vi "Remove Conditional Disable Structure.vi"(8 "error in (no error)":errorcluster, 11 "Assert VI Path":path) -> (0 "error out":errorcluster)   [LabVIEW 2018, in "Test.lvclass"]
uses:
  Test.lvclass
  <vilib>/Utility/traverseref.llb/TRef TravTarget.ctl
  Save VI Ref Source.ctl
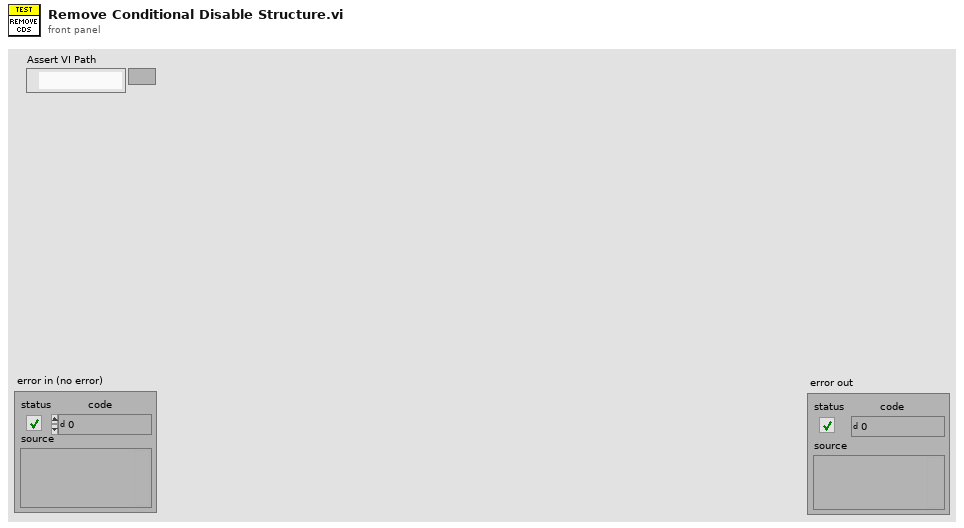
[diagram p1: front panel]
types:
  T1 = typedef "Save VI Ref Source.ctl" = enum16{"File Path", "VI Reference"}
  T2 = typedef "TRef TravTarget.ctl" = enum16{"FP", "BD", "Other"}
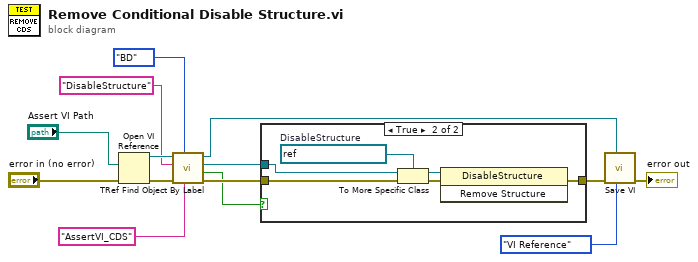
[diagram p0: block diagram]
diagram:
  n1 = Open VI Reference(vi path="Assert VI Path", error in (no error)="error in (no error)") -> (vi reference=w14:refnum<vi>, error out=w13:errorcluster)  [unwired: 4 in]
  n2 = call <vilib>:"TRef Find Object By Label.vi"("Label"="AssertVI_CDS" ("Class Name"), "Traverse Target"=TRef_TravTarget."BD", "error in (no error)"=w13, "Class Name"="DisableStructure", "VI Ref"=w14) -> ("error out"=w7:errorcluster, "Found?"=w6:bool, "Found Obj Ref"=w9:refnum<vi>, "dup VI Ref"=w4:refnum<vi>)  [unwired: 3 in]
  n3 = case shown="True" w6 {
    tunnel: w9 -> [_ w21]
    tunnel: w7 -> [w15 w19]
    tunnel: [w15 w16] -> w3
    frame False {
    }
    frame True {
      w20 = refnum<vi> refnum  # DisableStructure
      n4 = To More Specific Class(target class=w20, reference=w21, error in=w19) -> (specific class reference=w18:refnum<vi>, error out=w17:errorcluster)
      n5 = invoke class="DisableStructure" method="Remove Structure"(reference=w18, error in=w17) -> (error out=w16:errorcluster)  [unwired: 1 in, 2 out]
    }
  }
  n6 = call "Save VI.vi"("Reference Source"=Save_VI_Ref_Source."VI Reference", "VI Refnum"=w4, "error in (no error)"=w3) -> ("error out"=→"error out":errorcluster)  [unwired: 8 in]
